vi "from string array 1.0.vi"(8 "error in (no error)":errorcluster, 10 "String Array":string[][](array[string]), 11 "Multiplexer configuration in":refnum<class "Multiplexer configuration.lvclass">) -> (0 "error out":errorcluster, 3 "Multiplexer configuration out":refnum<class "Multiplexer configuration.lvclass">)   [LabVIEW 2021, in "Multiplexer configuration.lvclass"]
uses:
  Multiplexer configuration.lvclass
  <vilib>/NI/Tag Bus/tag/Data Type.ctl
  permissions.ctl
  Multiplexer configuration.lvclass/Multiplexer configuration.ctl
  Write Lines.vi
  Get Line Name.vi
  <vilib>/NI/Tag Bus Module Framework/module configuration/FindDuplicate.vi
  <vilib>/Utility/error.llb/Error Cluster From Error Code.vi
  <vilib>/NI/Tag Bus/tag/tag descriptor.lvclass
  <vilib>/NI/Tag Bus Module Framework/channel/TBM channel.lvclass
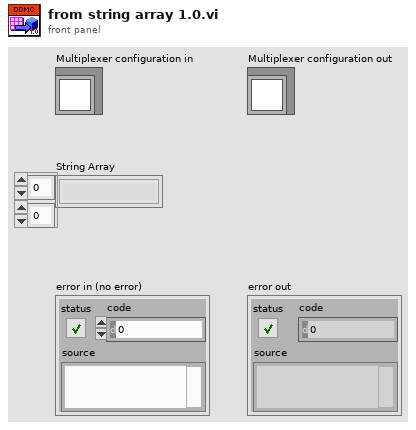
[diagram p1: front panel]
types:
  T1 = typedef "Multiplexer configuration.lvclass/permissions.ctl" = enum32{"Read from HW", "Write to HW"}
  T2 = typedef "tag bus.lvlib/tag descriptor.lvclass/Data Type.ctl" = enum16{"Double", "Single", "I64", "I32", "I16", "I8", "U64", "U32", "U16", "U8", "Boolean", "String", "Array of Double", "Array of Single", "Array of I64", "Array of I32", "Array of I16", "Array of I8", "Array of U64", "Array of U32", "Array of U16", "Array of U8", "Array of Boolean", "Array of String"}
  T3 = typedef "TBM channel.lvclass/channel classification.ctl" = enum16{"input data", "output data", "processing parameter", "processing result"}
  T4 = cluster{"[0]":refnum<class "TBM channel.lvclass">, "[1]":refnum<class "TBM channel.lvclass">, "[2]":refnum<class "TBM channel.lvclass">, "[3]":refnum<class "TBM channel.lvclass">}
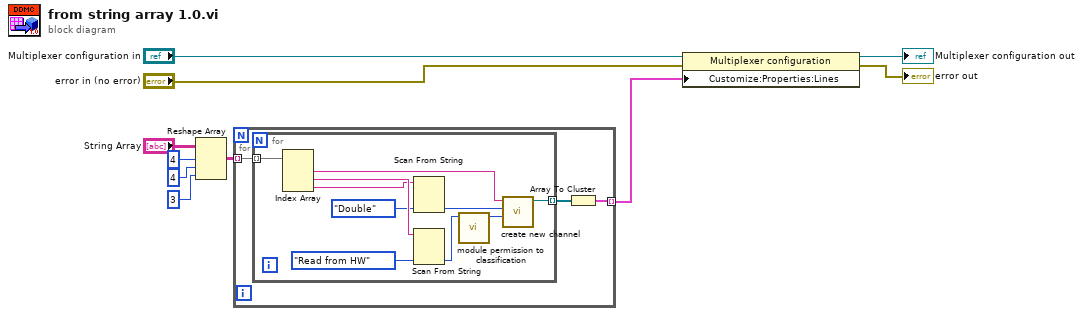
[diagram p0: block diagram]
diagram:
  n1 = Reshape Array("String Array", 4 ("dimension size"), 4 ("dimension size"), 3 ("dimension size")) -> (w5:string[][][])
  n2 = for {
    tunnel: w5 -> [w13] mode=indexing
    tunnel: [w11] -> w8 mode=indexing
    n3 = for {
      tunnel: w13 -> [w23] mode=indexing
      tunnel: [w14] -> w12 mode=indexing
      n4 = Index Array(array=w23) -> (element #1=w22:string, element #2=w21:string, element #3=w20:string)  [unwired: 3 in]
      n5 = Scan From String(input string=w20, default 1=Data_Type."Double" ("data type")) -> (output 1=w18:T2)  [unwired: 3 in, 3 out]
      n6 = Scan From String(input string=w21, default 1=permissions."Read from HW" ("view direction")) -> (output 1=w16:T1)  [unwired: 3 in, 3 out]
      n7 = call "module permission to classification.vi"("display permissions"=w16) -> ("channel classification"=w15:T3)  [unwired: 10 in]
      n8 = call <vilib>:"create new channel.vi"("channel classification"=w15, "data type"=w18, "channel name"=w22) -> ("channel"=w14:refnum<class "TBM channel.lvclass">)  [unwired: 8 in]
    }
    n9 = Array To Cluster(array=w12) -> (cluster=w11:T4)
  }
  n10 = property class="Multiplexer configuration"(reference="Multiplexer configuration in", error in="error in (no error)", "Customize:Properties:Lines"=w8) -> (reference out=→"Multiplexer configuration out":refnum<class "Multiplexer configuration.lvclass">, error out=→"error out":errorcluster)
